vi "增加用户.vi"(6 "用户名-refnum-in":refnum<vi>, 8 "用户类别-refnum-in":refnum<vi>, 9 "管理人员1+密码":string[][](array[string]), 10 "操作人员0+密码":string[][](array[string]), 11 "密码文件路径":path=path "E:/LabVIEW Data/盾构/default") -> (2 "管理人员1+密码_out":string[][](array[string]), 3 "操作人员0+密码_out":string[][](array[string]))   [LabVIEW 2018]
panel:
  out "用户名列表":i32(listbox)
  in  "请输入用户名":string
  in  "用户类别":u8(ring) caption="请在此选择用户类别" items=["操作人员", "管理人员"]
  in  "请输入密码":string
  in  "请输入新密码":string caption="请重新输入密码"
  in  "返回":bool
  in  "增加":bool
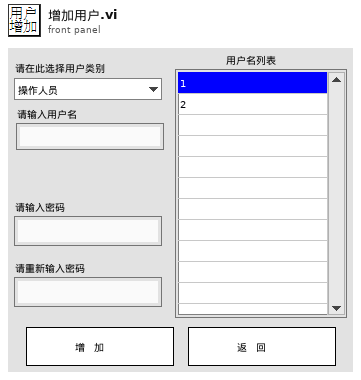
[diagram p1: front panel]
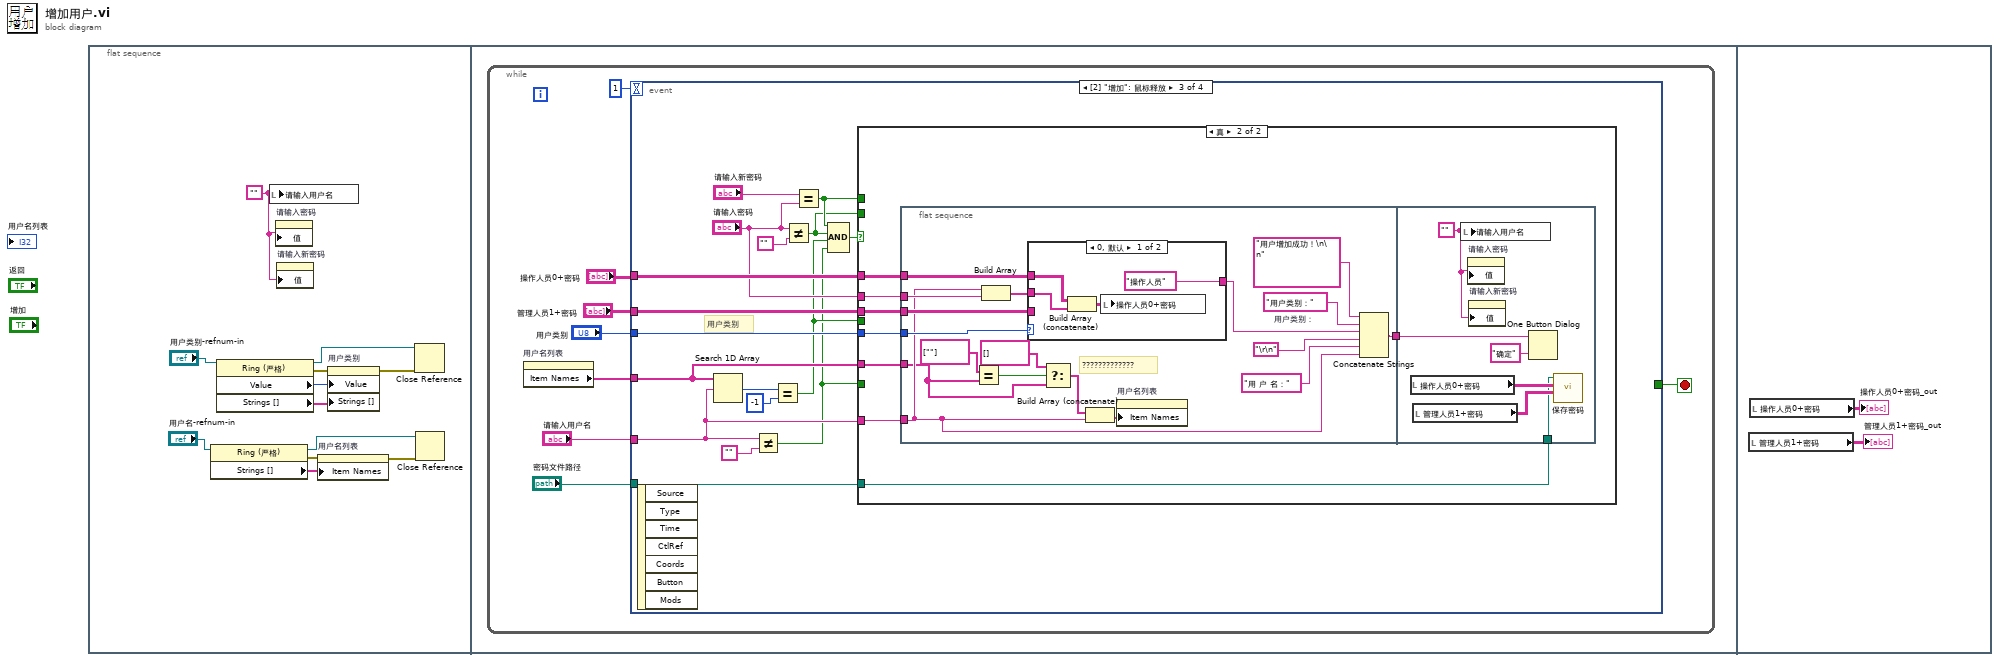
[diagram p0: block diagram]
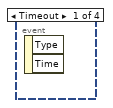
[diagram p2: hidden frame]
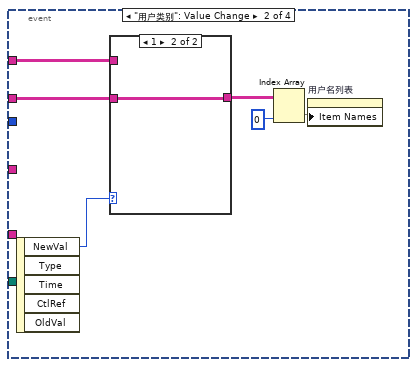
[diagram p3: hidden frame]
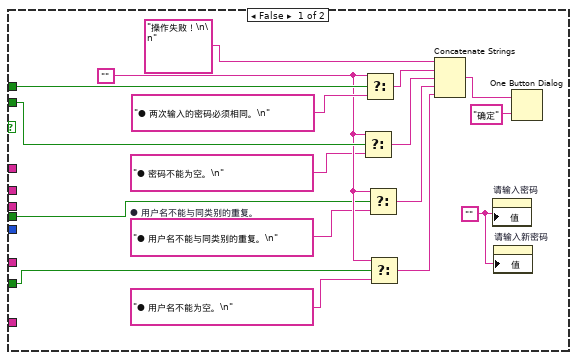
[diagram p5: hidden frame]
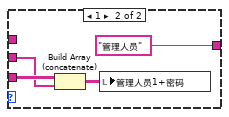
[diagram p6: hidden frame]
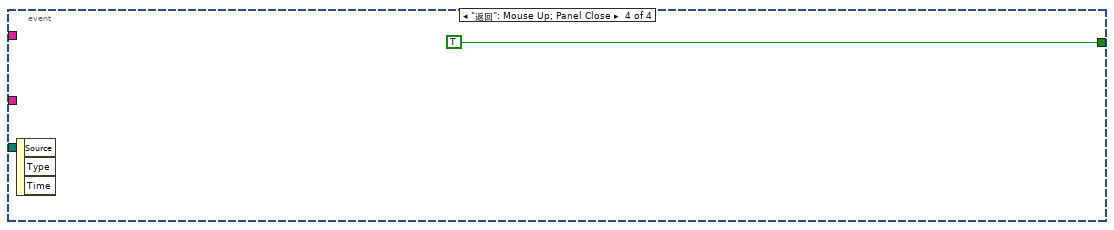
[diagram p7: hidden frame]
diagram:
  n1 = flat-sequence {
    frame #0 {
      w8 = ""
      n2 = property class="Ring (严格)"(reference="用户名-refnum-in") -> (reference out=w2:refnum<vi>, error out=w6:errorcluster, "Strings []"=w1:string[])  [unwired: 1 in]
      n3 = property class="Ring (严格)"(reference="用户类别-refnum-in") -> (reference out=w4:refnum<vi>, error out=w7:errorcluster, "Value"=w12:u8, "Strings []"=w10:string[])  [unwired: 1 in]
      n4 = local write "请输入用户名"(w8) -> ()
      n5 = property on="请输入密码" class="Str"("值"=w8) -> ()  [unwired: 2 in, 2 out]
      n6 = property on="请输入新密码" class="Str"("值"=w8) -> ()  [unwired: 2 in, 2 out]
      n7 = property on="用户名列表" class="LstBox (严格)"(error in=w6, "Item Names"=w1) -> (error out=w3:errorcluster)  [unwired: 1 in, 1 out]
      n8 = property on="用户类别" class="Ring (严格)"(error in=w7, "Value"=w12, "Strings []"=w10) -> (error out=w5:errorcluster)  [unwired: 1 in, 1 out]
      n9 = Close Reference(reference=w4, error in (no error)=w5) -> ()  [unwired: 1 out]
      n10 = Close Reference(reference=w2, error in (no error)=w3) -> ()  [unwired: 1 out]
    }
    frame #1 {
      n11 = while {
        stop <- w19 stop-if-true
        n12 = property on="用户名列表" class="LstBox (严格)"() -> ("Item Names"=w17:string[])  [unwired: 2 in, 2 out]
        n13 = event shown="[2] \"增加\": 鼠标释放" {
          selector: _ -> [_ _ _ _]
          dyn-events: _ -> [_ _ _ _]
          timeout: 1 -> [_ _ _ _]
          tunnel: "操作人员0+密码" -> [_ w23 w44 _]
          tunnel: "管理人员1+密码" -> [_ w24 w43 _]
          tunnel: "用户类别" -> [_ _ w45 _]
          tunnel: w17 -> [_ _ w41 _]
          tunnel: "密码文件路径" -> [_ _ w40 _]
          tunnel: [_ _ _ TRUE] -> w19
          tunnel: "请输入用户名" -> [_ _ w42 _]
          event Timeout {
            n14 = event-data() -> ()  [unwired: 1 in, 2 out]
          }
          event "用户类别": Value Change {
            n15 = event-data() -> ("NewVal"=w25:u8)  [unwired: 1 in, 4 out]
            n16 = case shown="1" w25 {
              tunnel: w23 -> [w27 _]
              tunnel: [w27 w28] -> w22
              tunnel: w24 -> [_ w28]
              frame 0, Default {
              }
              frame 1 {
              }
            }
            n17 = Index Array(array=w22, index (col)=0 ("禁用的索引 (col)")) -> (element=w21:string[])  [unwired: 1 in]
            n18 = property on="用户名列表" class="LstBox (严格)"("Item Names"=w21) -> ()  [unwired: 2 in, 2 out]
          }
          event "增加": Mouse Up {
            # "用户类别"
            n19 = event-data() -> ()  [unwired: 1 in, 7 out]
            n20 = Search 1D Array(1D array=w41, element=w42) -> (index of element=w35:i32)  [unwired: 1 in]
            n21 = Not Equal?(x=w42, y="") -> (x != y?=w29:bool)
            n22 = Equal?(x=w35, y=-1) -> (x = y?=w30:bool)
            n23 = Not Equal?(x="请输入密码", y="") -> (x != y?=w31:bool)
            n24 = Equal?(x="请输入新密码", y="请输入密码") -> (x = y?=w32:bool)
            n25 = Compound Arithmetic op=AND(w32, w31, w30, w29) -> (w37:bool)
            n26 = case shown="真" w37 {
              tunnel: w45 -> [_ w70]
              tunnel: w44 -> [_ w69]
              tunnel: w43 -> [_ w68]
              tunnel: w42 -> [_ w66]
              tunnel: w41 -> [_ w67]
              tunnel: "请输入密码" -> [_ w65]
              tunnel: w40 -> [_ w64]
              tunnel: w32 -> [w61 _]
              tunnel: w31 -> [w58 _]
              tunnel: w30 -> [w54 _]
              tunnel: w29 -> [w53 _]
              frame False {
                w55 = "● 用户名不能与同类别的重复。\n"  # ● 用户名不能与同类别的重复。
                w57 = ""
                w62 = ""
                n27 = Select(t=w57, s=w58, f="● 密码不能为空。\n") -> (s? t:f=w50:string)
                n28 = Select(t=w57, s=w61, f="● 两次输入的密码必须相同。\n") -> (s? t:f=w51:string)
                n29 = Select(t=w57, s=w54, f=w55) -> (s? t:f=w49:string)
                n30 = Select(t=w57, s=w53, f="● 用户名不能为空。\n") -> (s? t:f=w48:string)
                n31 = Concatenate Strings("操作失败！\n\n", w51, w50, w49, w48) -> (w47:string)
                n32 = property on="请输入密码" class="Str"("值"=w62) -> ()  [unwired: 2 in, 2 out]
                n33 = property on="请输入新密码" class="Str"("值"=w62) -> ()  [unwired: 2 in, 2 out]
                n34 = One Button Dialog(message=w47, button name ("OK")="确定" ("按钮名称（“确定”）")) -> ()  [unwired: 1 out]
              }
              frame True {
                n35 = flat-sequence {
                  tunnel: w70 -> [w88]
                  tunnel: w69 -> [w87]
                  tunnel: w68 -> [w86]
                  tunnel: w67 -> [w73]
                  tunnel: w66 -> [w77]
                  tunnel: w65 -> [w84]
                  tunnel: [w76] -> w63
                  tunnel: w64 -> [w100]
                  tunnel: w63 -> [w98]
                  frame #0 {
                    w82 = "用户类别："  # 用户类别：
                    # "?????????????"
                    n36 = Equal?(x=string[] [""] ("t"), y=w73) -> (x = y?=w74:bool)
                    n37 = Build Array(w77, w84) -> (w83:string[])
                    n38 = case shown="0, 默认" w88 {
                      tunnel: w86 -> [_ w96]
                      tunnel: w87 -> [w92 _]
                      tunnel: w83 -> [w91 w95]
                      tunnel: ["操作人员" "管理人员"] -> w81
                      frame 0, Default {
                        n39 = Build Array (concatenate)(w92, w91) -> (w90:string[][])
                        n40 = local write "操作人员0+密码"(w90) -> ()
                      }
                      frame 1 {
                        n41 = Build Array (concatenate)(w96, w95) -> (w94:string[][])
                        n42 = local write "管理人员1+密码"(w94) -> ()
                      }
                    }
                    n43 = Select(t=string[] [], s=w74, f=w73) -> (s? t:f=w71:string[])
                    n44 = Build Array (concatenate)(w71, w77) -> (w85:string[])
                    n45 = property on="用户名列表" class="LstBox (严格)"("Item Names"=w85) -> ()  [unwired: 2 in, 2 out]
                    n46 = Concatenate Strings("用户增加成功！\n\n", w82, w81, "\r\n", "用 户 名：", w77) -> (w76:string)
                  }
                  frame #1 {
                    w97 = ""
                    n47 = local read "操作人员0+密码"() -> (w102:string[][])
                    n48 = local read "管理人员1+密码"() -> (w101:string[][])
                    n49 = local write "请输入用户名"(w97) -> ()
                    n50 = property on="请输入密码" class="Str"("值"=w97) -> ()  [unwired: 2 in, 2 out]
                    n51 = property on="请输入新密码" class="Str"("值"=w97) -> ()  [unwired: 2 in, 2 out]
                    n52 = One Button Dialog(message=w98, button name ("OK")="确定" ("按钮名称（“确定”）")) -> ()  [unwired: 1 out]
                    n53 = call "保存密码.vi"("密码文件路径"=w100, "操作人员0+密码"=w102, "管理人员1+密码"=w101) -> ()  [unwired: 4 in, 1 out]
                  }
                }
              }
            }
          }
          event "返回": Mouse Up; Panel Close {
            n54 = event-data() -> ()  [unwired: 1 in, 3 out]
          }
        }
      }
    }
    frame #2 {
      n55 = local read "管理人员1+密码"() -> (→"管理人员1+密码_out":string[][])
      n56 = local read "操作人员0+密码"() -> (→"操作人员0+密码_out":string[][])
    }
  }
